vi "license file.vi"(1 "year":u16=2005) -> (0 "Accepted":bool)   [LabVIEW 2015]
uses:
  DAC project/Calibration and Function folders.ctl
  <vilib>/Utility/config.llb/Read Key (Boolean).vi
  <vilib>/Utility/config.llb/Write Key (Boolean).vi
  <vilib>/Utility/config.llb/NI_LVConfig.lvlib
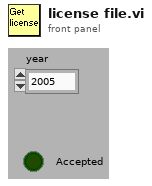
[diagram p1: front panel]
types:
  T1 = typedef "Calibration and Function folders.ctl" = enum16{"Sensors", "Functions", "Config File", "UserAppFolder"}
  T2 = typedef "NI_LVConfig.lvlib/Config Data RefNum.ctl" = refnum<k1>
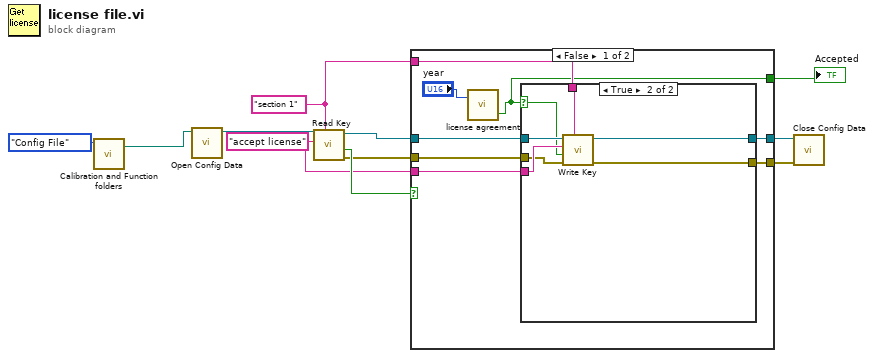
[diagram p0: block diagram]
diagram:
  w7 = "section 1" ("section")
  w8 = "accept license" ("key")
  n1 = call "Calibration and Function folders.vi"("Folder"=Calibration_and_Function_folders."Config File") -> ("Selected Folder"=w1:path)  [unwired: 10 in]
  n2 = call <vilib>:"Open Config Data.vi"("configuration file path"=w1) -> ("refnum"=w11:T2)  [unwired: 8 in, 2 out]
  n3 = call-poly <vilib>:"Read Key.vi"("section"=w7, "key"=w8, "refnum"=w11) -> ("error out"=w4:errorcluster, "value"=w10:bool, "refnum out"=w9:T2)  [unwired: 5 in, 1 out]
  n4 = case shown="False" w10 {
    selector: w10 -> [_ w29]
    tunnel: w9 -> [w18 w31]
    tunnel: w8 -> [w17 _]
    tunnel: w7 -> [w16 _]
    tunnel: [w15 w31] -> w6
    tunnel: [w14 w30] -> w5
    tunnel: w4 -> [w13 w30]
    tunnel: [w12 w29] -> w3
    frame False {
      n5 = call "license agreement.vi"("year"="year") -> ("Accepted"=w12:bool)  [unwired: 1 in, 1 out]
      n6 = case shown="True" w12 {
        selector: w12 -> [_ w26]
        tunnel: w18 -> [w21 w28]
        tunnel: w17 -> [_ w27]
        tunnel: w16 -> [_ w25]
        tunnel: [w21 w24] -> w15
        tunnel: [w20 w23] -> w14
        tunnel: w13 -> [w20 w22]
        frame False {
        }
        frame True {
          n7 = call-poly <vilib>:"Write Key.vi"("section"=w25, "error in (no error)"=w22, "value"=w26, "key"=w27, "refnum"=w28) -> ("error out"=w23:errorcluster, "refnum out"=w24:T2)  [unwired: 4 in, 1 out]
        }
      }
    }
    frame True {
    }
  }
  "Accepted" <- w3
  n8 = call <vilib>:"Close Config Data.vi"("error in (no error)"=w5, "refnum"=w6) -> ()  [unwired: 8 in, 2 out]
